vi "LSX Save Config.vi"(8 "error in (no error)":errorcluster, 10 "pcFileName":string, 11 "lLSID":i32) -> (0 "error out":errorcluster, 2 "pcFileName out":string, 3 "function return":i32)   [LabVIEW 2016, in "Tango_DLL.lvlib"]
doc: "TANGOAPI int TANGOCALL LSX_SaveConfig (int lLSID, char *pcFileName);"
uses:
  Tango_DLL.lvlib
  2017/Microscope Control/Device Library/Stages/Marzhauser/SCAN IM 120 x 80/Tango DLL VIs/Tango_DLL.dll
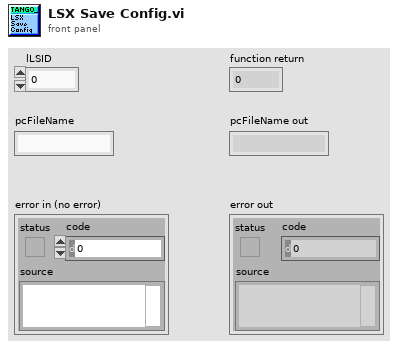
[diagram p1: front panel]
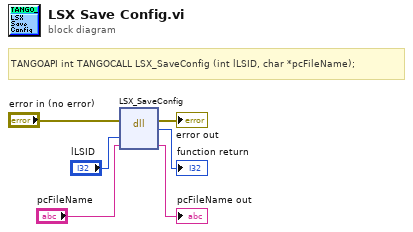
[diagram p0: block diagram]
diagram:
  # "TANGOAPI int TANGOCALL LSX_SaveConfig (int lLSID, char *pcFileName);"
  n1 = dll-call lib="C:/Users/4PiSMS/Documents/Microscope Control/2017/Microscope Control/Device Library/Stages/Marzhauser/SCAN IM 120 x 80/Tango DLL VIs/Tango_DLL.*" fn="LSX_SaveConfig"(error in="error in (no error)", "lLSID"="lLSID", "pcFileName"="pcFileName") -> (error out=→"error out":errorcluster, →"function return":i32, "pcFileName"=→"pcFileName out":string)  [unwired: 3 in, 1 out]
